vi "QCP_ReadFile.vi"(6 "Overrite Existing Data?":bool=TRUE, 8 "error in":errorcluster, 9 "Path Relative?":bool, 10 "Path":string, 11 "QCP_DevRef_In":T1) -> (0 "error out":errorcluster, 3 "QCP_DevRef_Out":T1)   [LabVIEW 2016]
uses:
  <userlib>/836-libraries/System/QCP_V2/QCPSupportCode/QCP_RefNum.ctl
  <userlib>/836-libraries/System/QCP_V2/QCPSupportCode/QCPData.ctl
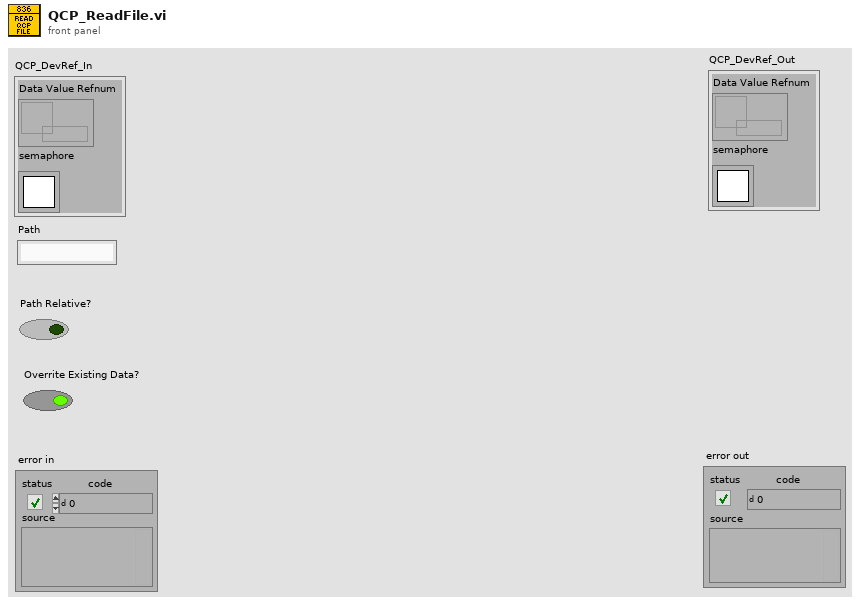
[diagram p1: front panel]
types:
  T1 = typedef "QCP_RefNum.ctl" = cluster{"Data Value Refnum":refnum<data-value>, "semaphore":T2}
  T2 = typedef "Semaphore RefNum" = refnum<k1>
  T3 = typedef "QCPData.ctl" = cluster{"Names":string[], "Values":cluster{"Array":dbl[]}[], "TuningMode?":bool}
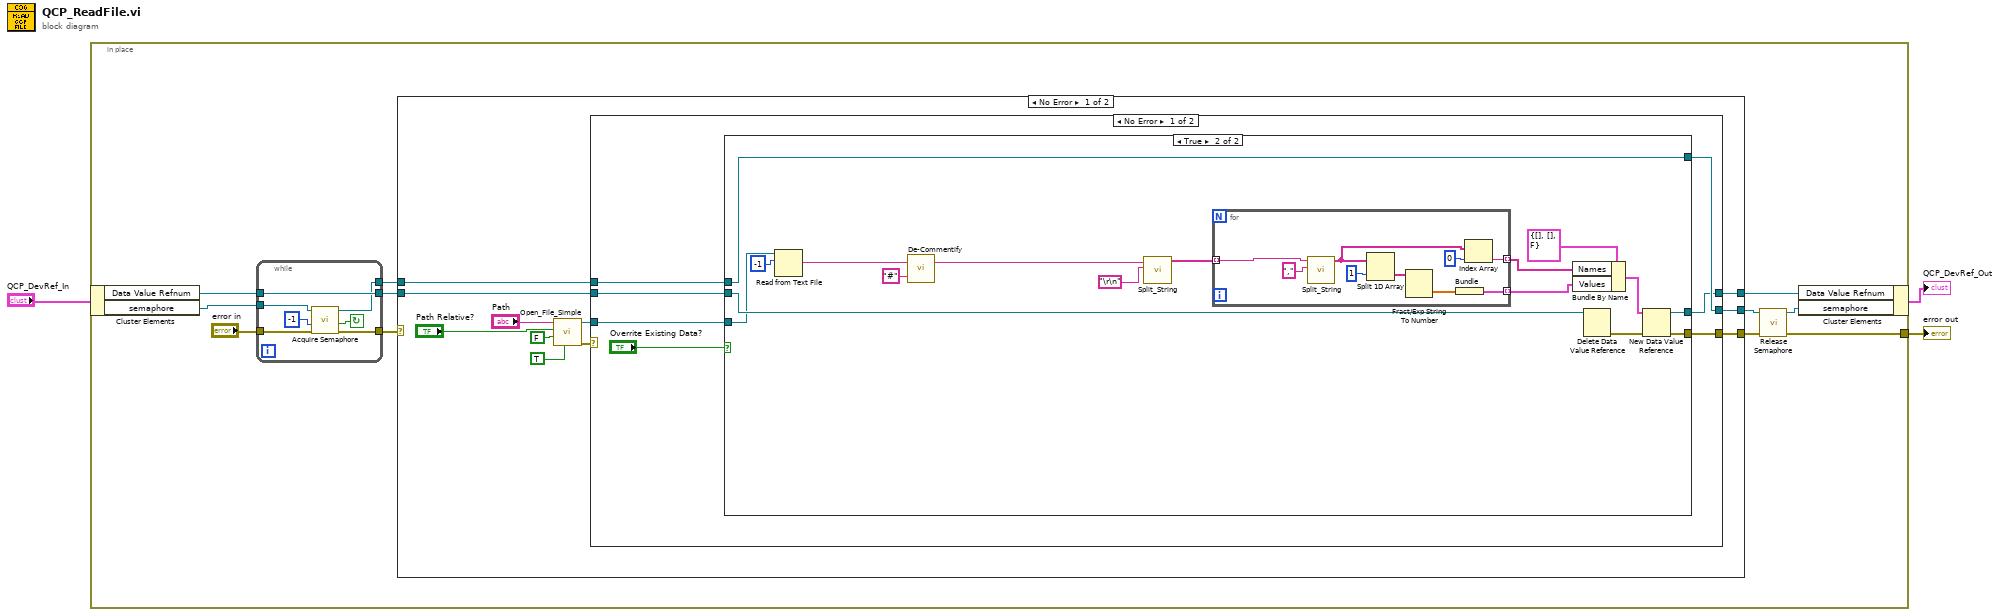
[diagram p0: block diagram]
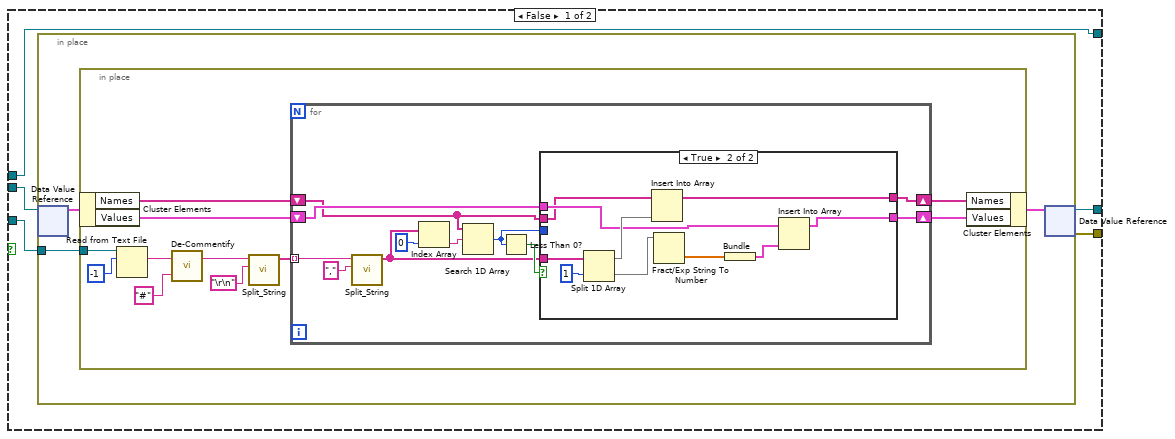
[diagram p2: hidden frame]
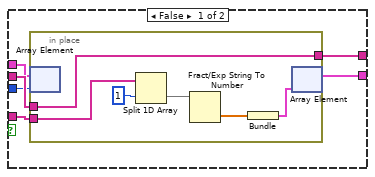
[diagram p3: hidden frame]
diagram:
  n1 = in-place {
    in-place-border: [w6] -> w1
    n2 = in-place-cluster #1("QCP_DevRef_In") -> ("Data Value Refnum"=w13:refnum<data-value>, "semaphore"=w14:T2)
    n3 = while {
      tunnel: w14 -> [w122]
      tunnel: [w119] -> w10
      tunnel: w13 -> [w119]
      tunnel: "error in" -> [w118]
      tunnel: [w117] -> w11
      tunnel: [w116] -> w9
      stop <- w121 continue-if-true
      n4 = call <vilib>:"Acquire Semaphore.vi"("error in (no error)"=w118, "ms timeout (-1)"=-1, "semaphore"=w122) -> ("error out"=w117:errorcluster, "timed out"=w121:bool, "semaphore out"=w116:T2)  [unwired: 2 in]
    }
    n5 = case shown="No Error" w11 {
      selector: w11 -> [_ w115]
      tunnel: [w21 w115] -> w7
      tunnel: w10 -> [w19 w114]
      tunnel: w9 -> [w16 w113]
      tunnel: [w18 w114] -> w5
      tunnel: [w15 w113] -> w4
      frame No Error {
        n6 = call <userlib>:"Open_File_Simple.vi"("Read Only?"=TRUE, "Overwrite?"=FALSE, "Path relative?"="Path Relative?", "Path"="Path") -> ("error out"=w22:errorcluster, "refnum out"=w17:refnum<file>)  [unwired: 6 in]
        n7 = case shown="No Error" w22 {
          selector: w22 -> [_ w112]
          tunnel: [w29 w112] -> w21
          tunnel: w19 -> [w31 w111]
          tunnel: [w26 w111] -> w18
          tunnel: w17 -> [w30 _]
          tunnel: w16 -> [w28 w110]
          tunnel: [w27 w110] -> w15
          frame No Error {
            n8 = case shown="True" "Overrite Existing Data?" {
              tunnel: w31 -> [w37 w100]
              tunnel: [w35 w99] -> w26
              tunnel: w30 -> [w36 w98]
              tunnel: [w34 w89] -> w29
              tunnel: [w33 w88] -> w27
              tunnel: w28 -> [w33 w88]
              frame False {
                n9 = in-place {
                  in-place-border: w36 -> [w38]
                  n10 = in-place-dvr #2(w37) -> (w40:T3)  [unwired: 1 out]
                  n11 = in-place {
                    in-place-border: w38 -> [w51]
                    n12 = in-place-cluster #3(w40) -> ("Names"=w47:string[], "Values"=w46:cluster{"Array":dbl[]}[])
                    n13 = Read from Text File(file (use dialog)=w51, count=-1) -> (text=w43:string)  [unwired: 2 in, 3 out]
                    n14 = call <userlib>:"De-Commentify.vi"("Comment Token"="#", "File Text"=w43) -> ("Text Out"=w42:string)  [unwired: 1 out]
                    n15 = call <userlib>:"Split_String.vi"("Delim Char"="\r\n", "Text In"=w42) -> ("Splits Out"=w48:string[])  [unwired: 8 in, 1 out]
                    n16 = for {
                      tunnel: w48 -> [w62] mode=indexing
                      shift-right: [w54] -> w45
                      shift-left: w47 -> [w55]
                      shift-right: [w53] -> w44
                      shift-left: w46 -> [w56]
                      n17 = call <userlib>:"Split_String.vi"("Delim Char"=",", "Text In"=w62) -> ("Splits Out"=w57:string[])  [unwired: 8 in, 1 out]
                      n18 = Index Array(array=w57, index=0) -> (element=w58:string)
                      n19 = Search 1D Array(1D array=w55, element=w58) -> (index of element=w52:i32)  [unwired: 1 in]
                      n20 = Less Than 0?(x=w52) -> (x < 0?=w59:bool)
                      n21 = case shown="True" w59 {
                        tunnel: w57 -> [w64 w84]
                        tunnel: w56 -> [w66 w78]
                        tunnel: [w63 w77] -> w53
                        tunnel: w55 -> [w67 w76]
                        tunnel: [w68 w75] -> w54
                        tunnel: w52 -> [w65 _]
                        frame False {
                          n22 = in-place {
                            in-place-border: [w74] -> w68
                            in-place-border: w67 -> [w74]
                            in-place-border: w64 -> [w73]
                            n23 = in-place-array #4(w66, w65) -> ()  [unwired: 1 out]
                            n24 = Split 1D Array(array=w73, index=1) -> (second subarray=w71:string[])  [unwired: 1 out]
                            n25 = Fract/Exp String To Number(string=w71) -> (number=w70:dbl[])  [unwired: 3 in, 1 out]
                            n26 = Bundle(w70) -> (w69:cluster{dbl[]})  [unwired: 1 in]
                            n27 = in-place-array #4(w69) -> (w63:cluster{"Array":dbl[]}[])  [unwired: 1 out]
                          }
                        }
                        frame True {
                          n28 = Split 1D Array(array=w84, index=1) -> (first subarray=w81:string[], second subarray=w82:string[])
                          n29 = Insert Into Array(array=w76, new element=w81) -> (w75:string[])  [unwired: 1 in]
                          n30 = Fract/Exp String To Number(string=w82) -> (number=w80:dbl[])  [unwired: 3 in, 1 out]
                          n31 = Bundle(w80) -> (w79:cluster{dbl[]})  [unwired: 1 in]
                          n32 = Insert Into Array(array=w78, new element=w79) -> (w77:cluster{"Array":dbl[]}[])  [unwired: 1 in]
                        }
                      }
                    }
                    n33 = in-place-cluster #3("Names"=w45, "Values"=w44) -> (w39:T3)
                  }
                  n34 = in-place-dvr #2(w39) -> (w35:refnum<data-value>, w34:errorcluster)
                }
              }
              frame True {
                n35 = Read from Text File(file (use dialog)=w98, count=-1) -> (text=w87:string)  [unwired: 2 in, 3 out]
                n36 = call <userlib>:"De-Commentify.vi"("Comment Token"="#", "File Text"=w87) -> ("Text Out"=w85:string)  [unwired: 1 out]
                n37 = call <userlib>:"Split_String.vi"("Delim Char"="\r\n", "Text In"=w85) -> ("Splits Out"=w95:string[])  [unwired: 8 in, 1 out]
                n38 = for {
                  tunnel: w95 -> [w109] mode=indexing
                  tunnel: [w102] -> w92 mode=indexing
                  tunnel: [w101] -> w93 mode=indexing
                  n39 = call <userlib>:"Split_String.vi"("Delim Char"=",", "Text In"=w109) -> ("Splits Out"=w106:string[])  [unwired: 8 in, 1 out]
                  n40 = Split 1D Array(array=w106, index=1) -> (second subarray=w104:string[])  [unwired: 1 out]
                  n41 = Fract/Exp String To Number(string=w104) -> (number=w103:dbl[])  [unwired: 3 in, 1 out]
                  n42 = Bundle(w103) -> (w102:cluster{dbl[]})  [unwired: 1 in]
                  n43 = Index Array(array=w106, index=0) -> (element=w101:string)
                }
                n44 = Bundle By Name(cluster=T3 {"Names"=[], "Values"=[], "TuningMode?"=FALSE} ("QCP Data Ref"), "Names"=w93, "Values"=w92) -> (w91:T3)
                n45 = Delete Data Value Reference(data value reference=w100) -> (error out=w90:errorcluster)  [unwired: 1 in, 1 out]
                n46 = New Data Value Reference(data value=w91, error in=w90) -> (data value reference=w99:refnum<data-value>, error out=w89:errorcluster)
              }
            }
          }
          frame Error {
          }
        }
      }
      frame Error {
      }
    }
    n47 = call <vilib>:"Release Semaphore.vi"("error in (no error)"=w7, "semaphore"=w4) -> ("error out"=w6:errorcluster, "semaphore out"=w8:T2)  [unwired: 4 in]
    n48 = in-place-cluster #1("Data Value Refnum"=w5, "semaphore"=w8) -> (→"QCP_DevRef_Out":T1)
  }
  "error out" <- w1
